vi "S4GUI_003.vi"(7 "Tab ObsEng":enum32{"Obs", "CCD modes", "Guider", "Eng"}(tab)) -> ()   [LabVIEW 2018] (continued)
            n1971 = local write "P15"(w3878) -> ()
            n1972 = call-dynamic "Write sequencia_ant.vi"("error in (no error)"=w3873, "sequencia_ant"=w3869, "Opt_Selector in"=w3875) -> ("error out"=w3872:errorcluster, "Opt_Selector out"=w3874:refnum<class "Opt_Selector.lvclass">)  [unwired: 7 in]
          }
          frame 2 {
            w3882 = u16 15 ("sequencia")
            w3891 = FALSE ("P0")
            w3892 = FALSE ("P0")
            w3893 = FALSE ("P0")
            w3894 = TRUE ("P0")
            # "0000 0000 0000 1111 = 15"
            n1973 = local write "P0"(w3894) -> ()
            n1974 = local write "P1"(w3894) -> ()
            n1975 = local write "P2"(w3894) -> ()
            n1976 = local write "P3"(w3894) -> ()
            n1977 = local write "P4"(w3892) -> ()
            n1978 = local write "P5"(w3892) -> ()
            n1979 = local write "P6"(w3892) -> ()
            n1980 = local write "P7"(w3892) -> ()
            n1981 = call-dynamic "Write sequencia.vi"("error in (no error)"=w3889, "sequencia"=w3882, "Opt_Selector in"=w3890) -> ("error out"=w3886:errorcluster, "Opt_Selector out"=w3888:refnum<class "Opt_Selector.lvclass">)  [unwired: 7 in]
            n1982 = call-dynamic "Write sequencia_ant.vi"("error in (no error)"=w3886, "sequencia_ant"=w3882, "Opt_Selector in"=w3888) -> ("error out"=w3885:errorcluster, "Opt_Selector out"=w3887:refnum<class "Opt_Selector.lvclass">)  [unwired: 7 in]
            n1983 = local write "P8"(w3893) -> ()
            n1984 = local write "P9"(w3893) -> ()
            n1985 = local write "P10"(w3893) -> ()
            n1986 = local write "P11"(w3893) -> ()
            n1987 = local write "P12"(w3891) -> ()
            n1988 = local write "P13"(w3891) -> ()
            n1989 = local write "P14"(w3891) -> ()
            n1990 = local write "P15"(w3891) -> ()
          }
          frame 3 {
            w3895 = u16 3855 ("sequencia")
            w3904 = FALSE ("P0")
            w3905 = FALSE ("P0")
            w3906 = TRUE ("P0")
            w3907 = TRUE ("P0")
            # "0000 1111 0000 1111 = 3855"
            n1991 = local write "P0"(w3907) -> ()
            n1992 = local write "P1"(w3907) -> ()
            n1993 = local write "P2"(w3907) -> ()
            n1994 = local write "P3"(w3907) -> ()
            n1995 = local write "P4"(w3905) -> ()
            n1996 = local write "P5"(w3905) -> ()
            n1997 = local write "P6"(w3905) -> ()
            n1998 = local write "P7"(w3905) -> ()
            n1999 = call-dynamic "Write sequencia.vi"("error in (no error)"=w3902, "sequencia"=w3895, "Opt_Selector in"=w3903) -> ("error out"=w3900:errorcluster, "Opt_Selector out"=w3901:refnum<class "Opt_Selector.lvclass">)  [unwired: 7 in]
            n2000 = local write "P8"(w3906) -> ()
            n2001 = local write "P9"(w3906) -> ()
            n2002 = local write "P10"(w3906) -> ()
            n2003 = local write "P11"(w3906) -> ()
            n2004 = local write "P12"(w3904) -> ()
            n2005 = local write "P13"(w3904) -> ()
            n2006 = local write "P14"(w3904) -> ()
            n2007 = local write "P15"(w3904) -> ()
            n2008 = call-dynamic "Write sequencia_ant.vi"("error in (no error)"=w3900, "sequencia_ant"=w3895, "Opt_Selector in"=w3901) -> ("error out"=w3899:errorcluster, "Opt_Selector out"=w3898:refnum<class "Opt_Selector.lvclass">)  [unwired: 7 in]
          }
          frame 4 {
            w3908 = u16 0 ("sequencia")
            w3917 = FALSE ("P0")
            w3918 = FALSE ("P0")
            w3919 = FALSE ("P0")
            w3920 = FALSE ("P0")
            n2009 = local write "P0"(w3920) -> ()
            n2010 = local write "P1"(w3920) -> ()
            n2011 = local write "P2"(w3920) -> ()
            n2012 = local write "P3"(w3920) -> ()
            n2013 = local write "P4"(w3918) -> ()
            n2014 = local write "P5"(w3918) -> ()
            n2015 = local write "P6"(w3918) -> ()
            n2016 = local write "P7"(w3918) -> ()
            n2017 = call-dynamic "Write sequencia.vi"("error in (no error)"=w3915, "sequencia"=w3908, "Opt_Selector in"=w3916) -> ("error out"=w3912:errorcluster, "Opt_Selector out"=w3914:refnum<class "Opt_Selector.lvclass">)  [unwired: 7 in]
            n2018 = call-dynamic "Write sequencia_ant.vi"("error in (no error)"=w3912, "sequencia_ant"=w3908, "Opt_Selector in"=w3914) -> ("error out"=w3911:errorcluster, "Opt_Selector out"=w3913:refnum<class "Opt_Selector.lvclass">)  [unwired: 7 in]
            n2019 = local write "P8"(w3919) -> ()
            n2020 = local write "P9"(w3919) -> ()
            n2021 = local write "P10"(w3919) -> ()
            n2022 = local write "P11"(w3919) -> ()
            n2023 = local write "P12"(w3917) -> ()
            n2024 = local write "P13"(w3917) -> ()
            n2025 = local write "P14"(w3917) -> ()
            n2026 = local write "P15"(w3917) -> ()
          }
          frame 5 {
            n2027 = call-dynamic "Read sequencia_ant.vi"("error in (no error)"=w3924, "Opt_Selector in"=w3925) -> ("error out"=w3923:errorcluster, "sequencia_ant"=w3921:u16, "Opt_Selector out"=w3922:refnum<class "Opt_Selector.lvclass">)  [unwired: 7 in]
          }
        }
        n2028 = call "Write WPROT.vi"("error in (no error)"=w3817, "Opt_Selector.lvclass"=w3824, "Instrument in"=w3823) -> ("error out"=w3826:errorcluster, "Instrument out"=w3827:refnum<class "Instrument.lvclass">)  [unwired: 7 in]
        n2029 = property on="#Pol. Seq. Done" class="Slide (strict)"(error in=w3817, "Scale.Maximum"=w3818, "Scale.Minimum"=w3816) -> ()  [unwired: 1 in, 2 out]
        n2030 = call "Write Instrument.lvclass.vi"("error in (no error)"=w3826, "Instrument.lvclass"=w3827, "S4ACS_GUI in"=w3822) -> ("error out"=w3806:errorcluster, "S4ACS_GUI out"=w3807:refnum<class "S4GUI.lvclass">)  [unwired: 7 in]
        n2031 = call "Read Instrument.lvclass.vi"("error in (no error)"=w3806, "S4ACS_GUI in"=w3807) -> ("error out"=w3811:errorcluster, "Instrument.lvclass"=w3812:refnum<class "Instrument.lvclass">, "S4ACS_GUI out"=w3815:refnum<class "S4GUI.lvclass">)  [unwired: 7 in]
        n2032 = call "Read ASEL.vi"("error in (no error)"=w3811, "Instrument in"=w3812) -> ("error out"=w3803:errorcluster, "Opt_Selector.lvclass"=w3805:refnum<class "Opt_Selector.lvclass">, "Instrument out"=w3808:refnum<class "Instrument.lvclass">)  [unwired: 7 in]
        n2033 = call "Read name_pos.vi"("error in (no error)"=w3803, "Optics in"=w3805) -> ("error out"=w3802:errorcluster, "name_pos"=w3801:string, "Optics out"=w3804:refnum<class "Opt_Selector.lvclass">)  [unwired: 7 in]
        n2034 = call "Write ASEL.vi"("error in (no error)"=w3802, "Opt_Selector.lvclass"=w3804, "Instrument in"=w3808) -> ("error out"=w3809:errorcluster, "Instrument out"=w3813:refnum<class "Instrument.lvclass">)  [unwired: 7 in]
        n2035 = case shown="\"ON\"" w3801 {
          tunnel: w3809 -> [w3832 w3843]
          tunnel: [w3832 w3839] -> w3810
          tunnel: w3813 -> [w3831 w3844]
          tunnel: [w3831 w3840] -> w3814
          frame Default {
          }
          frame "ON" {
            n2036 = call "Read WPROT.vi"("error in (no error)"=w3843, "Instrument in"=w3844) -> ("error out"=w3835:errorcluster, "Opt_Selector.lvclass"=w3842:refnum<class "Opt_Selector.lvclass">, "Instrument out"=w3841:refnum<class "Instrument.lvclass">)  [unwired: 7 in]
            n2037 = call-dynamic "Read sequencia.vi"("error in (no error)"=w3835, "Opt_Selector in"=w3842) -> ("error out"=w3834:errorcluster, "sequencia"=w3838:u16, "Opt_Selector out"=w3837:refnum<class "Opt_Selector.lvclass">)  [unwired: 7 in]
            n2038 = case shown="0" w3838 {
              tunnel: w3837 -> [w3846 w3855]
              tunnel: [w3846 w3851] -> w3836
              tunnel: w3834 -> [w3845 w3854]
              tunnel: [w3845 w3849] -> w3833
              frame Default {
              }
              frame 0 {
                n2039 = call-dynamic "Write sequencia.vi"("error in (no error)"=w3854, "sequencia"=u16 1, "Opt_Selector in"=w3855) -> ("error out"=w3850:errorcluster, "Opt_Selector out"=w3852:refnum<class "Opt_Selector.lvclass">)  [unwired: 7 in]
                n2040 = local write "P0"(TRUE ("P0")) -> ()
                n2041 = call-dynamic "Write sequencia_ant.vi"("error in (no error)"=w3850, "sequencia_ant"=u16 1, "Opt_Selector in"=w3852) -> ("error out"=w3849:errorcluster, "Opt_Selector out"=w3851:refnum<class "Opt_Selector.lvclass">)  [unwired: 7 in]
              }
            }
            n2042 = call "Write WPROT.vi"("error in (no error)"=w3833, "Opt_Selector.lvclass"=w3836, "Instrument in"=w3841) -> ("error out"=w3839:errorcluster, "Instrument out"=w3840:refnum<class "Instrument.lvclass">)  [unwired: 7 in]
          }
        }
        n2043 = call "Write Instrument.lvclass.vi"("error in (no error)"=w3810, "Instrument.lvclass"=w3814, "S4ACS_GUI in"=w3815) -> ("error out"=w3738:errorcluster, "S4ACS_GUI out"=w3739:refnum<class "S4GUI.lvclass">)  [unwired: 7 in]
        n2044 = call-dynamic "Read AcquisitionA.vi"("error in (no error)"=w3738, "S4ACS_GUI in"=w3739) -> ("error out"=w3798:errorcluster, "Acquisition.lvclass"=w3800:refnum<class "Acquisition.lvclass">, "S4ACS_GUI out"=w3797:refnum<class "S4GUI.lvclass">)  [unwired: 7 in]
        n2045 = call-dynamic "Read Channel.vi"("error in (no error)"=w3798, "Acquisition in"=w3800) -> ("error out"=w3794:errorcluster, "Channel.lvclass"=w3795:refnum<class "Channel.lvclass">, "Acquisition out"=w3799:refnum<class "Acquisition.lvclass">)  [unwired: 7 in]
        n2046 = call-dynamic "Write sequencias.vi"("error in (no error)"=w3794, "sequencias"=w3742, "Channel in"=w3795) -> ("error out"=w3791:errorcluster, "Channel out"=w3793:refnum<class "Channel.lvclass">)  [unwired: 7 in]
        n2047 = call-dynamic "Write prev sequencias.vi"("error in (no error)"=w3791, "prev sequencias"=w3742, "Channel in"=w3793) -> ("error out"=w3790:errorcluster, "Channel out"=w3792:refnum<class "Channel.lvclass">)  [unwired: 7 in]
        n2048 = call-dynamic "Write Channel.vi"("error in (no error)"=w3790, "Channel.lvclass"=w3792, "Acquisition in"=w3799) -> ("error out"=w3789:errorcluster, "Acquisition out"=w3796:refnum<class "Acquisition.lvclass">)  [unwired: 7 in]
        n2049 = call-dynamic "Write AcquisitionA.vi"("error in (no error)"=w3789, "Acquisition.lvclass"=w3796, "S4ACS_GUI in"=w3797) -> ("error out"=w3747:errorcluster, "S4ACS_GUI out"=w3748:refnum<class "S4GUI.lvclass">)  [unwired: 7 in]
        n2050 = call "Read AcquisitionB.vi"("error in (no error)"=w3747, "S4ACS_GUI in"=w3748) -> ("error out"=w3774:errorcluster, "Acquisition.lvclass"=w3776:refnum<class "Acquisition.lvclass">, "S4ACS_GUI out"=w3773:refnum<class "S4GUI.lvclass">)  [unwired: 7 in]
        n2051 = call-dynamic "Read Channel.vi"("error in (no error)"=w3774, "Acquisition in"=w3776) -> ("error out"=w3770:errorcluster, "Channel.lvclass"=w3771:refnum<class "Channel.lvclass">, "Acquisition out"=w3775:refnum<class "Acquisition.lvclass">)  [unwired: 7 in]
        n2052 = call-dynamic "Write sequencias.vi"("error in (no error)"=w3770, "sequencias"=w3742, "Channel in"=w3771) -> ("error out"=w3767:errorcluster, "Channel out"=w3769:refnum<class "Channel.lvclass">)  [unwired: 7 in]
        n2053 = call-dynamic "Write prev sequencias.vi"("error in (no error)"=w3767, "prev sequencias"=w3742, "Channel in"=w3769) -> ("error out"=w3766:errorcluster, "Channel out"=w3768:refnum<class "Channel.lvclass">)  [unwired: 7 in]
        n2054 = call-dynamic "Write Channel.vi"("error in (no error)"=w3766, "Channel.lvclass"=w3768, "Acquisition in"=w3775) -> ("error out"=w3765:errorcluster, "Acquisition out"=w3772:refnum<class "Acquisition.lvclass">)  [unwired: 7 in]
        n2055 = call "Write AcquisitionB.vi"("error in (no error)"=w3765, "Acquisition.lvclass"=w3772, "S4ACS_GUI in"=w3773) -> ("error out"=w3749:errorcluster, "S4ACS_GUI out"=w3750:refnum<class "S4GUI.lvclass">)  [unwired: 7 in]
        n2056 = call-dynamic "Read AcquisitionC.vi"("error in (no error)"=w3749, "S4ACS_GUI in"=w3750) -> ("error out"=w3762:errorcluster, "Acquisition.lvclass"=w3764:refnum<class "Acquisition.lvclass">, "S4ACS_GUI out"=w3761:refnum<class "S4GUI.lvclass">)  [unwired: 7 in]
        n2057 = call-dynamic "Read Channel.vi"("error in (no error)"=w3762, "Acquisition in"=w3764) -> ("error out"=w3758:errorcluster, "Channel.lvclass"=w3759:refnum<class "Channel.lvclass">, "Acquisition out"=w3763:refnum<class "Acquisition.lvclass">)  [unwired: 7 in]
        n2058 = call-dynamic "Write sequencias.vi"("error in (no error)"=w3758, "sequencias"=w3742, "Channel in"=w3759) -> ("error out"=w3755:errorcluster, "Channel out"=w3757:refnum<class "Channel.lvclass">)  [unwired: 7 in]
        n2059 = call-dynamic "Write prev sequencias.vi"("error in (no error)"=w3755, "prev sequencias"=w3742, "Channel in"=w3757) -> ("error out"=w3754:errorcluster, "Channel out"=w3756:refnum<class "Channel.lvclass">)  [unwired: 7 in]
        n2060 = call-dynamic "Write Channel.vi"("error in (no error)"=w3754, "Channel.lvclass"=w3756, "Acquisition in"=w3763) -> ("error out"=w3753:errorcluster, "Acquisition out"=w3760:refnum<class "Acquisition.lvclass">)  [unwired: 7 in]
        n2061 = call-dynamic "Write AcquisitionC.vi"("error in (no error)"=w3753, "Acquisition.lvclass"=w3760, "S4ACS_GUI in"=w3761) -> ("error out"=w3745:errorcluster, "S4ACS_GUI out"=w3746:refnum<class "S4GUI.lvclass">)  [unwired: 7 in]
        n2062 = call-dynamic "Read AcquisitionD.vi"("error in (no error)"=w3745, "S4ACS_GUI in"=w3746) -> ("error out"=w3786:errorcluster, "Acquisition.lvclass"=w3788:refnum<class "Acquisition.lvclass">, "S4ACS_GUI out"=w3785:refnum<class "S4GUI.lvclass">)  [unwired: 7 in]
        n2063 = call-dynamic "Read Channel.vi"("error in (no error)"=w3786, "Acquisition in"=w3788) -> ("error out"=w3782:errorcluster, "Channel.lvclass"=w3783:refnum<class "Channel.lvclass">, "Acquisition out"=w3787:refnum<class "Acquisition.lvclass">)  [unwired: 7 in]
        n2064 = call-dynamic "Write sequencias.vi"("error in (no error)"=w3782, "sequencias"=w3742, "Channel in"=w3783) -> ("error out"=w3779:errorcluster, "Channel out"=w3781:refnum<class "Channel.lvclass">)  [unwired: 7 in]
        n2065 = call-dynamic "Write prev sequencias.vi"("error in (no error)"=w3779, "prev sequencias"=w3742, "Channel in"=w3781) -> ("error out"=w3778:errorcluster, "Channel out"=w3780:refnum<class "Channel.lvclass">)  [unwired: 7 in]
        n2066 = call-dynamic "Write Channel.vi"("error in (no error)"=w3778, "Channel.lvclass"=w3780, "Acquisition in"=w3787) -> ("error out"=w3777:errorcluster, "Acquisition out"=w3784:refnum<class "Acquisition.lvclass">)  [unwired: 7 in]
        n2067 = call-dynamic "Write AcquisitionD.vi"("error in (no error)"=w3777, "Acquisition.lvclass"=w3784, "S4ACS_GUI in"=w3785) -> ("error out"=w3743:errorcluster, "S4ACS_GUI out"=w3744:refnum<class "S4GUI.lvclass">)  [unwired: 7 in]
        n2068 = call-dynamic "Write sequencias.vi"("error in (no error)"=w3743, "sequencias"=w3742, "S4GUI in"=w3744) -> ("error out"=w3752:errorcluster, "S4GUI out"=w3751:refnum<class "S4GUI.lvclass">)  [unwired: 7 in]
        n2069 = call-dynamic "Write prev sequencias.vi"("error in (no error)"=w3752, "prev sequencias"=w3742, "S4GUI in"=w3751) -> ("error out"=w3740:errorcluster, "S4GUI out"=w3741:refnum<class "S4GUI.lvclass">)  [unwired: 7 in]
      }
      event "P0", "P1", "P2", "P3", "P4", "P5", "P6", "P7", "P8", "P9", "P10", "P11", "P12", "P13", "P14", "P15": Value Change {
        w4041 = u16 5 items=["All 16 positions", "First 8 positions", "First 4 positions", "0-3 + 8-11", "Clear", "Customized"] ("Select Positions")
        # "Garantir que, quando em POLARIMETRIA, pelo menos WP1 esteja selecionado."
        # "Salva tambem em \nSequencia_ant para\no caso de repeticao."
        n2070 = event-data() -> ()  [unwired: 1 in, 6 out]
        n2071 = local write "Select Positions"(w4041) -> ()
        n2072 = call "Read Instrument.lvclass.vi"("error in (no error)"=w4023, "S4ACS_GUI in"=w4024) -> ("error out"=w4018:errorcluster, "Instrument.lvclass"=w4021:refnum<class "Instrument.lvclass">, "S4ACS_GUI out"=w4022:refnum<class "S4GUI.lvclass">)  [unwired: 7 in]
        n2073 = Build Array("P0", "P1", "P2", "P3", "P4", "P5", "P6", "P7", "P8", "P9", "P10", "P11", "P12", "P13", "P14", "P15") -> (w4010:bool[])
        n2074 = call "Read WPROT.vi"("error in (no error)"=w4018, "Instrument in"=w4021) -> ("error out"=w4017:errorcluster, "Opt_Selector.lvclass"=w4019:refnum<class "Opt_Selector.lvclass">, "Instrument out"=w4020:refnum<class "Instrument.lvclass">)  [unwired: 7 in]
        n2075 = Boolean Array To Number(Boolean array=w4010) -> (number=w4025:u32)
        n2076 = To Unsigned Word Integer(number=w4025) -> (unsigned 16bit integer=w3928:u16)
        n2077 = call-dynamic "Write sequencia.vi"("error in (no error)"=w4017, "sequencia"=w3928, "Opt_Selector in"=w4019) -> ("error out"=w4012:errorcluster, "Opt_Selector out"=w4014:refnum<class "Opt_Selector.lvclass">)  [unwired: 7 in]
        n2078 = call-dynamic "Write sequencia_ant.vi"("error in (no error)"=w4012, "sequencia_ant"=w3928, "Opt_Selector in"=w4014) -> ("error out"=w4011:errorcluster, "Opt_Selector out"=w4013:refnum<class "Opt_Selector.lvclass">)  [unwired: 7 in]
        n2079 = call "Write WPROT.vi"("error in (no error)"=w4011, "Opt_Selector.lvclass"=w4013, "Instrument in"=w4020) -> ("error out"=w4016:errorcluster, "Instrument out"=w4015:refnum<class "Instrument.lvclass">)  [unwired: 7 in]
        n2080 = call "Write Instrument.lvclass.vi"("error in (no error)"=w4016, "Instrument.lvclass"=w4015, "S4ACS_GUI in"=w4022) -> ("error out"=w3991:errorcluster, "S4ACS_GUI out"=w3992:refnum<class "S4GUI.lvclass">)  [unwired: 7 in]
        n2081 = call "Read Instrument.lvclass.vi"("error in (no error)"=w3991, "S4ACS_GUI in"=w3992) -> ("error out"=w3997:errorcluster, "Instrument.lvclass"=w3996:refnum<class "Instrument.lvclass">, "S4ACS_GUI out"=w3993:refnum<class "S4GUI.lvclass">)  [unwired: 7 in]
        n2082 = call "Read ASEL.vi"("error in (no error)"=w3997, "Instrument in"=w3996) -> ("error out"=w4003:errorcluster, "Opt_Selector.lvclass"=w4001:refnum<class "Opt_Selector.lvclass">, "Instrument out"=w4000:refnum<class "Instrument.lvclass">)  [unwired: 7 in]
        n2083 = call "Read name_pos.vi"("error in (no error)"=w4003, "Optics in"=w4001) -> ("error out"=w4004:errorcluster, "name_pos"=w4005:string, "Optics out"=w4002:refnum<class "Opt_Selector.lvclass">)  [unwired: 7 in]
        n2084 = call "Write ASEL.vi"("error in (no error)"=w4004, "Opt_Selector.lvclass"=w4002, "Instrument in"=w4000) -> ("error out"=w3999:errorcluster, "Instrument out"=w3995:refnum<class "Instrument.lvclass">)  [unwired: 7 in]
        n2085 = case shown="\"ON\"" w4005 {
          tunnel: w3999 -> [w4043 w4054]
          tunnel: [w4043 w4050] -> w3998
          tunnel: w3995 -> [w4042 w4055]
          tunnel: [w4042 w4051] -> w3994
          frame Default {
          }
          frame "ON" {
            n2086 = call "Read WPROT.vi"("error in (no error)"=w4054, "Instrument in"=w4055) -> ("error out"=w4046:errorcluster, "Opt_Selector.lvclass"=w4053:refnum<class "Opt_Selector.lvclass">, "Instrument out"=w4052:refnum<class "Instrument.lvclass">)  [unwired: 7 in]
            n2087 = call-dynamic "Read sequencia.vi"("error in (no error)"=w4046, "Opt_Selector in"=w4053) -> ("error out"=w4045:errorcluster, "sequencia"=w4049:u16, "Opt_Selector out"=w4048:refnum<class "Opt_Selector.lvclass">)  [unwired: 7 in]
            n2088 = case shown="0" w4049 {
              tunnel: w4048 -> [w4057 w4066]
              tunnel: [w4057 w4062] -> w4047
              tunnel: w4045 -> [w4056 w4065]
              tunnel: [w4056 w4060] -> w4044
              frame Default {
              }
              frame 0 {
                n2089 = call-dynamic "Write sequencia.vi"("error in (no error)"=w4065, "sequencia"=u16 1, "Opt_Selector in"=w4066) -> ("error out"=w4061:errorcluster, "Opt_Selector out"=w4063:refnum<class "Opt_Selector.lvclass">)  [unwired: 7 in]
                n2090 = local write "P0"(TRUE ("P0")) -> ()
                n2091 = call-dynamic "Write sequencia_ant.vi"("error in (no error)"=w4061, "sequencia_ant"=u16 1, "Opt_Selector in"=w4063) -> ("error out"=w4060:errorcluster, "Opt_Selector out"=w4062:refnum<class "Opt_Selector.lvclass">)  [unwired: 7 in]
              }
            }
            n2092 = call "Write WPROT.vi"("error in (no error)"=w4044, "Opt_Selector.lvclass"=w4047, "Instrument in"=w4052) -> ("error out"=w4050:errorcluster, "Instrument out"=w4051:refnum<class "Instrument.lvclass">)  [unwired: 7 in]
          }
        }
        n2093 = for {
          tunnel: w4010 -> [w4070] mode=indexing
          shift-right: [w4069] -> w4008
          shift-left: 0 -> [w4067]
          # "calcula qtd de 1s"
          n2094 = Increment(x=w4067) -> (x+1=w4068:i32)
          n2095 = Select(t=w4068, s=w4070, f=w4067) -> (s? t:f=w4069:i32)
        }
        n2096 = property on="#Pol. Seq. Done" class="Slide (strict)"("Scale.Maximum"=w4008, "Scale.Minimum"=0.0 ("Scale.Range:Minimum")) -> ()  [unwired: 2 in, 2 out]
        n2097 = call "Write Instrument.lvclass.vi"("error in (no error)"=w3998, "Instrument.lvclass"=w3994, "S4ACS_GUI in"=w3993) -> ("error out"=w3935:errorcluster, "S4ACS_GUI out"=w3936:refnum<class "S4GUI.lvclass">)  [unwired: 7 in]
        n2098 = call-dynamic "Read AcquisitionA.vi"("error in (no error)"=w3935, "S4ACS_GUI in"=w3936) -> ("error out"=w3988:errorcluster, "Acquisition.lvclass"=w3990:refnum<class "Acquisition.lvclass">, "S4ACS_GUI out"=w3987:refnum<class "S4GUI.lvclass">)  [unwired: 7 in]
        n2099 = call-dynamic "Read Channel.vi"("error in (no error)"=w3988, "Acquisition in"=w3990) -> ("error out"=w3984:errorcluster, "Channel.lvclass"=w3985:refnum<class "Channel.lvclass">, "Acquisition out"=w3989:refnum<class "Acquisition.lvclass">)  [unwired: 7 in]
        n2100 = call-dynamic "Write sequencias.vi"("error in (no error)"=w3984, "sequencias"=w3928, "Channel in"=w3985) -> ("error out"=w3981:errorcluster, "Channel out"=w3983:refnum<class "Channel.lvclass">)  [unwired: 7 in]
        n2101 = call-dynamic "Write prev sequencias.vi"("error in (no error)"=w3981, "prev sequencias"=w3928, "Channel in"=w3983) -> ("error out"=w3980:errorcluster, "Channel out"=w3982:refnum<class "Channel.lvclass">)  [unwired: 7 in]
        n2102 = call-dynamic "Write Channel.vi"("error in (no error)"=w3980, "Channel.lvclass"=w3982, "Acquisition in"=w3989) -> ("error out"=w3979:errorcluster, "Acquisition out"=w3986:refnum<class "Acquisition.lvclass">)  [unwired: 7 in]
        n2103 = call-dynamic "Write AcquisitionA.vi"("error in (no error)"=w3979, "Acquisition.lvclass"=w3986, "S4ACS_GUI in"=w3987) -> ("error out"=w3933:errorcluster, "S4ACS_GUI out"=w3934:refnum<class "S4GUI.lvclass">)  [unwired: 7 in]
        n2104 = call "Read AcquisitionB.vi"("error in (no error)"=w3933, "S4ACS_GUI in"=w3934) -> ("error out"=w3964:errorcluster, "Acquisition.lvclass"=w3966:refnum<class "Acquisition.lvclass">, "S4ACS_GUI out"=w3963:refnum<class "S4GUI.lvclass">)  [unwired: 7 in]
        n2105 = call-dynamic "Read Channel.vi"("error in (no error)"=w3964, "Acquisition in"=w3966) -> ("error out"=w3960:errorcluster, "Channel.lvclass"=w3961:refnum<class "Channel.lvclass">, "Acquisition out"=w3965:refnum<class "Acquisition.lvclass">)  [unwired: 7 in]
        n2106 = call-dynamic "Write sequencias.vi"("error in (no error)"=w3960, "sequencias"=w3928, "Channel in"=w3961) -> ("error out"=w3957:errorcluster, "Channel out"=w3959:refnum<class "Channel.lvclass">)  [unwired: 7 in]
        n2107 = call-dynamic "Write prev sequencias.vi"("error in (no error)"=w3957, "prev sequencias"=w3928, "Channel in"=w3959) -> ("error out"=w3956:errorcluster, "Channel out"=w3958:refnum<class "Channel.lvclass">)  [unwired: 7 in]
        n2108 = call-dynamic "Write Channel.vi"("error in (no error)"=w3956, "Channel.lvclass"=w3958, "Acquisition in"=w3965) -> ("error out"=w3955:errorcluster, "Acquisition out"=w3962:refnum<class "Acquisition.lvclass">)  [unwired: 7 in]
        n2109 = call "Write AcquisitionB.vi"("error in (no error)"=w3955, "Acquisition.lvclass"=w3962, "S4ACS_GUI in"=w3963) -> ("error out"=w3937:errorcluster, "S4ACS_GUI out"=w3938:refnum<class "S4GUI.lvclass">)  [unwired: 7 in]
        n2110 = call-dynamic "Read AcquisitionC.vi"("error in (no error)"=w3937, "S4ACS_GUI in"=w3938) -> ("error out"=w3952:errorcluster, "Acquisition.lvclass"=w3954:refnum<class "Acquisition.lvclass">, "S4ACS_GUI out"=w3951:refnum<class "S4GUI.lvclass">)  [unwired: 7 in]
        n2111 = call-dynamic "Read Channel.vi"("error in (no error)"=w3952, "Acquisition in"=w3954) -> ("error out"=w3948:errorcluster, "Channel.lvclass"=w3949:refnum<class "Channel.lvclass">, "Acquisition out"=w3953:refnum<class "Acquisition.lvclass">)  [unwired: 7 in]
        n2112 = call-dynamic "Write sequencias.vi"("error in (no error)"=w3948, "sequencias"=w3928, "Channel in"=w3949) -> ("error out"=w3945:errorcluster, "Channel out"=w3947:refnum<class "Channel.lvclass">)  [unwired: 7 in]
        n2113 = call-dynamic "Write prev sequencias.vi"("error in (no error)"=w3945, "prev sequencias"=w3928, "Channel in"=w3947) -> ("error out"=w3944:errorcluster, "Channel out"=w3946:refnum<class "Channel.lvclass">)  [unwired: 7 in]
        n2114 = call-dynamic "Write Channel.vi"("error in (no error)"=w3944, "Channel.lvclass"=w3946, "Acquisition in"=w3953) -> ("error out"=w3943:errorcluster, "Acquisition out"=w3950:refnum<class "Acquisition.lvclass">)  [unwired: 7 in]
        n2115 = call-dynamic "Write AcquisitionC.vi"("error in (no error)"=w3943, "Acquisition.lvclass"=w3950, "S4ACS_GUI in"=w3951) -> ("error out"=w3931:errorcluster, "S4ACS_GUI out"=w3932:refnum<class "S4GUI.lvclass">)  [unwired: 7 in]
        n2116 = call-dynamic "Read AcquisitionD.vi"("error in (no error)"=w3931, "S4ACS_GUI in"=w3932) -> ("error out"=w3976:errorcluster, "Acquisition.lvclass"=w3978:refnum<class "Acquisition.lvclass">, "S4ACS_GUI out"=w3975:refnum<class "S4GUI.lvclass">)  [unwired: 7 in]
        n2117 = call-dynamic "Read Channel.vi"("error in (no error)"=w3976, "Acquisition in"=w3978) -> ("error out"=w3972:errorcluster, "Channel.lvclass"=w3973:refnum<class "Channel.lvclass">, "Acquisition out"=w3977:refnum<class "Acquisition.lvclass">)  [unwired: 7 in]
        n2118 = call-dynamic "Write sequencias.vi"("error in (no error)"=w3972, "sequencias"=w3928, "Channel in"=w3973) -> ("error out"=w3969:errorcluster, "Channel out"=w3971:refnum<class "Channel.lvclass">)  [unwired: 7 in]
        n2119 = call-dynamic "Write prev sequencias.vi"("error in (no error)"=w3969, "prev sequencias"=w3928, "Channel in"=w3971) -> ("error out"=w3968:errorcluster, "Channel out"=w3970:refnum<class "Channel.lvclass">)  [unwired: 7 in]
        n2120 = call-dynamic "Write Channel.vi"("error in (no error)"=w3968, "Channel.lvclass"=w3970, "Acquisition in"=w3977) -> ("error out"=w3967:errorcluster, "Acquisition out"=w3974:refnum<class "Acquisition.lvclass">)  [unwired: 7 in]
        n2121 = call-dynamic "Write AcquisitionD.vi"("error in (no error)"=w3967, "Acquisition.lvclass"=w3974, "S4ACS_GUI in"=w3975) -> ("error out"=w3929:errorcluster, "S4ACS_GUI out"=w3930:refnum<class "S4GUI.lvclass">)  [unwired: 7 in]
        n2122 = call-dynamic "Write sequencias.vi"("error in (no error)"=w3929, "sequencias"=w3928, "S4GUI in"=w3930) -> ("error out"=w3941:errorcluster, "S4GUI out"=w3940:refnum<class "S4GUI.lvclass">)  [unwired: 7 in]
        n2123 = call-dynamic "Write prev sequencias.vi"("error in (no error)"=w3941, "prev sequencias"=w3928, "S4GUI in"=w3940) -> ("error out"=w3942:errorcluster, "S4GUI out"=w3939:refnum<class "S4GUI.lvclass">)  [unwired: 7 in]
      }
      event "SSM": Value Change {
        # "F: fotom.\nT: polar."
        n2124 = event-data() -> ("NewVal"=w4078:u16)  [unwired: 1 in, 5 out]
        n2125 = call-dynamic "Read mode EXPOSE.vi"("error in (no error)"=w4084, "S4GUI in"=w4085) -> ("error out"=w4083:errorcluster, "mode EXPOSE"=w4079:bool, "S4GUI out"=w4080:refnum<class "S4GUI.lvclass">)  [unwired: 7 in]
        n2126 = call "Read Instrument.lvclass.vi"("error in (no error)"=w4083, "S4ACS_GUI in"=w4080) -> ("error out"=w4082:errorcluster, "Instrument.lvclass"=w4088:refnum<class "Instrument.lvclass">, "S4ACS_GUI out"=w4087:refnum<class "S4GUI.lvclass">)  [unwired: 7 in]
        n2127 = call-dynamic "Read mode.vi"("error in (no error)"=w4082, "Instrument in"=w4088) -> ("error out"=w4081:errorcluster, "mode"=w4086:bool)  [unwired: 7 in, 1 out]
        n2128 = case shown="1" w4078 {
          tunnel: [TRUE FALSE] -> w4091
          tunnel: w4081 -> [w4102 w4328]
          tunnel: w4087 -> [w4104 w4327]
          tunnel: [w4095 w4319] -> w4090
          tunnel: [w4094 w4318] -> w4089
          tunnel: w4086 -> [_ w4308]
          tunnel: w4079 -> [_ w4306]
          tunnel: ["SYNCHRONOUS" "ASYNCHRONOUS"] -> w4071
          frame 1 {
            # "Sync mode: Os canais sao configurados para Trigger externo, desde que o SyncBox esteja conectado."
            # "Sync by Cycle"
            n2129 = call-dynamic "Read Sync Box.lvclass.vi"("error in (no error)"=w4102, "SPARC4_AC in"=w4104) -> ("error out"=w4101:errorcluster, "Sync Box.lvclass"=w4105:refnum<class "Sync Box.lvclass">, "SPARC4_AC out"=w4103:refnum<class "S4GUI.lvclass">)  [unwired: 7 in]
            n2130 = call "Read connection.vi"("error in (no error)"=w4101, "Server in"=w4105) -> ("error out"=w4100:errorcluster, "connection"=w4099:bool)  [unwired: 7 in, 1 out]
            n2131 = case shown="False" w4099 {
              tunnel: [w4108 w4125] -> w4097
              tunnel: w4103 -> [w4108 w4115]
              tunnel: w4100 -> [w4107 w4114]
              tunnel: [w4107 w4109] -> w4096
              frame False {
              }
              frame True {
                n2132 = call-dynamic "Read AcquisitionC.vi"("error in (no error)"=w4114, "S4ACS_GUI in"=w4115) -> ("error out"=w4132:errorcluster, "Acquisition.lvclass"=w4131:refnum<class "Acquisition.lvclass">)  [unwired: 7 in, 1 out]
                n2133 = call-dynamic "Read AcquisitionA.vi"("error in (no error)"=w4114, "S4ACS_GUI in"=w4115) -> ("error out"=w4135:errorcluster, "Acquisition.lvclass"=w4136:refnum<class "Acquisition.lvclass">, "S4ACS_GUI out"=w4124:refnum<class "S4GUI.lvclass">)  [unwired: 7 in]
                n2134 = call "Read AcquisitionB.vi"("error in (no error)"=w4114, "S4ACS_GUI in"=w4115) -> ("error out"=w4133:errorcluster, "Acquisition.lvclass"=w4134:refnum<class "Acquisition.lvclass">)  [unwired: 7 in, 1 out]
                n2135 = call-dynamic "Read AcquisitionD.vi"("error in (no error)"=w4114, "S4ACS_GUI in"=w4115) -> ("error out"=w4129:errorcluster, "Acquisition.lvclass"=w4130:refnum<class "Acquisition.lvclass">)  [unwired: 7 in, 1 out]
                n2136 = call-dynamic "Read enabled.vi"("error in (no error)"=w4129, "Server in"=w4130) -> ("error out"=w4138:errorcluster, "enabled"=w4137:bool, "Server out"=w4139:refnum<class "Acquisition.lvclass">)  [unwired: 7 in]
                n2137 = call-dynamic "Read enabled.vi"("error in (no error)"=w4132, "Server in"=w4131) -> ("error out"=w4141:errorcluster, "enabled"=w4140:bool, "Server out"=w4142:refnum<class "Acquisition.lvclass">)  [unwired: 7 in]
                n2138 = call-dynamic "Read enabled.vi"("error in (no error)"=w4133, "Server in"=w4134) -> ("error out"=w4144:errorcluster, "enabled"=w4143:bool, "Server out"=w4145:refnum<class "Acquisition.lvclass">)  [unwired: 7 in]
                n2139 = call-dynamic "Read enabled.vi"("error in (no error)"=w4135, "Server in"=w4136) -> ("error out"=w4147:errorcluster, "enabled"=w4146:bool, "Server out"=w4148:refnum<class "Acquisition.lvclass">)  [unwired: 7 in]
                n2140 = case shown="True" w4143 {
                  tunnel: w4145 -> [w4228 w4232]
                  tunnel: w4144 -> [w4227 w4231]
                  tunnel: [w4228 w4230] -> w4121
                  tunnel: [w4227 w4229] -> w4120
                  frame False {
                  }
                  frame True {
                    # "Ext Start"
                    # "nome do arquivo .cfg"
                    # "seção no arquivo .cfg"
                    n2141 = call-dynamic "Read Channel.vi"("error in (no error)"=w4231, "Acquisition in"=w4232) -> ("error out"=w4236:errorcluster, "Channel.lvclass"=w4235:refnum<class "Channel.lvclass">, "Acquisition out"=w4234:refnum<class "Acquisition.lvclass">)  [unwired: 7 in]
                    n2142 = call-dynamic "Read Interface.vi"("error in (no error)"=w4236, "Channel in"=w4235) -> ("error out"=w4244:errorcluster, "Interface.lvclass"=w4245:refnum<class "Interface.lvclass">, "Channel out"=w4233:refnum<class "Channel.lvclass">)  [unwired: 7 in]
                    n2143 = call-dynamic "Get CCD_Config.vi"("error in (no error)"=w4244, "Interface in"=w4245) -> ("error out"=w4241:errorcluster, "output cluster"=w4240:T31, "Interface out"=w4246:refnum<class "Interface.lvclass">)  [unwired: 7 in]
                    n2144 = Bundle By Name(cluster=w4240, "TRIGGER_MODE"=u8 6 ("SHUTTER_MODE")) -> (w4242:T31)
                    n2145 = call-dynamic "Set CCD_Config.vi"("error in (no error)"=w4241, "input cluster"=w4242, "Interface in"=w4246) -> ("error out"=w4239:errorcluster, "Interface out"=w4247:refnum<class "Interface.lvclass">)  [unwired: 7 in]
                    n2146 = Flatten To String(anything=w4242, error in (no error)=w4239) -> (data string=w4237:string, error out=w4238:errorcluster)  [unwired: 2 in, 1 out]
                    n2147 = call "Write flatted cluster.vi"("error in (no error)"=w4238, "flatted cluster"=w4237, "Interface in"=w4247) -> ("error out"=w4249:errorcluster, "Interface out"=w4248:refnum<class "Interface.lvclass">)  [unwired: 7 in]
                    n2148 = call-dynamic "Write Interface.vi"("error in (no error)"=w4249, "Interface.lvclass"=w4248, "Channel in"=w4233) -> ("error out"=w4255:errorcluster, "Channel out"=w4256:refnum<class "Channel.lvclass">)  [unwired: 7 in]
                    n2149 = call "Write section_name.vi"("error in (no error)"=w4255, "section_name"="CCD_ACS2", "Channel in"=w4256) -> ("error out"=w4253:errorcluster, "Channel out"=w4259:refnum<class "Channel.lvclass">)  [unwired: 7 in]
                    n2150 = call-dynamic "save config.vi"("error in (no error)"=w4253, "file config"="lastsaved.cfg", "Channel in"=w4259) -> ("error out"=w4254:errorcluster, "Channel out"=w4260:refnum<class "Channel.lvclass">)  [unwired: 7 in]
                    n2151 = call-dynamic "Read State Machine.vi"("error in (no error)"=w4254, "Device in"=w4260) -> ("error out"=w4250:errorcluster, "State Machine.lvclass"=w4262:refnum<class "State Machine.lvclass">, "Device out"=w4261:refnum<class "Channel.lvclass">)  [unwired: 7 in]
                    n2152 = call-dynamic "Write State.vi"("error in (no error)"=w4250, "State"=60, "State Machine in"=w4262) -> ("error out"=w4251:errorcluster, "State Machine out"=w4263:refnum<class "State Machine.lvclass">)  [unwired: 7 in]
                    n2153 = call-dynamic "Write State Machine.vi"("error in (no error)"=w4251, "State Machine.lvclass"=w4263, "Device in"=w4261) -> ("error out"=w4265:errorcluster, "Device out"=w4264:refnum<class "Channel.lvclass">)  [unwired: 7 in]
                    n2154 = call-dynamic "Write Channel.vi"("error in (no error)"=w4265, "Channel.lvclass"=w4264, "Acquisition in"=w4234) -> ("error out"=w4229:errorcluster, "Acquisition out"=w4230:refnum<class "Acquisition.lvclass">)  [unwired: 7 in]
                  }
                }
                n2155 = case shown="True" w4146 {
                  tunnel: [w4266 w4300] -> w4122
                  tunnel: [w4267 w4299] -> w4123
                  tunnel: w4148 -> [w4267 w4269]
                  tunnel: w4147 -> [w4266 w4268]
                  frame False {
                  }
                  frame True {
                    # "nome do arquivo .cfg"
                    # "seção no arquivo .cfg"
                    # "Ext Start"
                    n2156 = call-dynamic "Read Channel.vi"("error in (no error)"=w4268, "Acquisition in"=w4269) -> ("error out"=w4301:errorcluster, "Channel.lvclass"=w4302:refnum<class "Channel.lvclass">, "Acquisition out"=w4303:refnum<class "Acquisition.lvclass">)  [unwired: 7 in]
                    n2157 = call-dynamic "Read Interface.vi"("error in (no error)"=w4301, "Channel in"=w4302) -> ("error out"=w4291:errorcluster, "Interface.lvclass"=w4290:refnum<class "Interface.lvclass">, "Channel out"=w4304:refnum<class "Channel.lvclass">)  [unwired: 7 in]
                    n2158 = call-dynamic "Get CCD_Config.vi"("error in (no error)"=w4291, "Interface in"=w4290) -> ("error out"=w4294:errorcluster, "output cluster"=w4295:T31, "Interface out"=w4289:refnum<class "Interface.lvclass">)  [unwired: 7 in]
                    n2159 = Bundle By Name(cluster=w4295, "TRIGGER_MODE"=u8 6 ("SHUTTER_MODE")) -> (w4293:T31)
                    n2160 = call-dynamic "Set CCD_Config.vi"("error in (no error)"=w4294, "input cluster"=w4293, "Interface in"=w4289) -> ("error out"=w4296:errorcluster, "Interface out"=w4288:refnum<class "Interface.lvclass">)  [unwired: 7 in]
                    n2161 = Flatten To String(anything=w4293, error in (no error)=w4296) -> (data string=w4298:string, error out=w4297:errorcluster)  [unwired: 2 in, 1 out]
                    n2162 = call "Write flatted cluster.vi"("error in (no error)"=w4297, "flatted cluster"=w4298, "Interface in"=w4288) -> ("error out"=w4286:errorcluster, "Interface out"=w4287:refnum<class "Interface.lvclass">)  [unwired: 7 in]
                    n2163 = call-dynamic "Write Interface.vi"("error in (no error)"=w4286, "Interface.lvclass"=w4287, "Channel in"=w4304) -> ("error out"=w4281:errorcluster, "Channel out"=w4280:refnum<class "Channel.lvclass">)  [unwired: 7 in]
                    n2164 = call "Write section_name.vi"("error in (no error)"=w4281, "section_name"="CCD_ACS1", "Channel in"=w4280) -> ("error out"=w4282:errorcluster, "Channel out"=w4277:refnum<class "Channel.lvclass">)  [unwired: 7 in]
                    n2165 = call-dynamic "save config.vi"("error in (no error)"=w4282, "file config"="lastsaved.cfg", "Channel in"=w4277) -> ("error out"=w4270:errorcluster, "Channel out"=w4271:refnum<class "Channel.lvclass">)  [unwired: 7 in]
                    n2166 = call-dynamic "Read State Machine.vi"("error in (no error)"=w4270, "Device in"=w4271) -> ("error out"=w4285:errorcluster, "State Machine.lvclass"=w4275:refnum<class "State Machine.lvclass">, "Device out"=w4276:refnum<class "Channel.lvclass">)  [unwired: 7 in]
                    n2167 = call-dynamic "Write State.vi"("error in (no error)"=w4285, "State"=60, "State Machine in"=w4275) -> ("error out"=w4284:errorcluster, "State Machine out"=w4274:refnum<class "State Machine.lvclass">)  [unwired: 7 in]
                    n2168 = call-dynamic "Write State Machine.vi"("error in (no error)"=w4284, "State Machine.lvclass"=w4274, "Device in"=w4276) -> ("error out"=w4272:errorcluster, "Device out"=w4273:refnum<class "Channel.lvclass">)  [unwired: 7 in]
                    n2169 = call-dynamic "Write Channel.vi"("error in (no error)"=w4272, "Channel.lvclass"=w4273, "Acquisition in"=w4303) -> ("error out"=w4300:errorcluster, "Acquisition out"=w4299:refnum<class "Acquisition.lvclass">)  [unwired: 7 in]
                  }
                }
                n2170 = case shown="True" w4140 {
                  tunnel: w4142 -> [w4189 w4193]
                  tunnel: w4141 -> [w4188 w4192]
                  tunnel: [w4189 w4191] -> w4119
                  tunnel: [w4188 w4190] -> w4118
                  frame False {
                  }
                  frame True {
                    # "Ext Start"
                    # "nome do arquivo .cfg"
                    # "seção no arquivo .cfg"
                    n2171 = call-dynamic "Read Channel.vi"("error in (no error)"=w4192, "Acquisition in"=w4193) -> ("error out"=w4197:errorcluster, "Channel.lvclass"=w4196:refnum<class "Channel.lvclass">, "Acquisition out"=w4195:refnum<class "Acquisition.lvclass">)  [unwired: 7 in]
                    n2172 = call-dynamic "Read Interface.vi"("error in (no error)"=w4197, "Channel in"=w4196) -> ("error out"=w4205:errorcluster, "Interface.lvclass"=w4206:refnum<class "Interface.lvclass">, "Channel out"=w4194:refnum<class "Channel.lvclass">)  [unwired: 7 in]
                    n2173 = call-dynamic "Get CCD_Config.vi"("error in (no error)"=w4205, "Interface in"=w4206) -> ("error out"=w4202:errorcluster, "output cluster"=w4201:T31, "Interface out"=w4207:refnum<class "Interface.lvclass">)  [unwired: 7 in]
                    n2174 = Bundle By Name(cluster=w4201, "TRIGGER_MODE"=u8 6 ("SHUTTER_MODE")) -> (w4203:T31)
                    n2175 = call-dynamic "Set CCD_Config.vi"("error in (no error)"=w4202, "input cluster"=w4203, "Interface in"=w4207) -> ("error out"=w4200:errorcluster, "Interface out"=w4208:refnum<class "Interface.lvclass">)  [unwired: 7 in]
                    n2176 = Flatten To String(anything=w4203, error in (no error)=w4200) -> (data string=w4198:string, error out=w4199:errorcluster)  [unwired: 2 in, 1 out]
                    n2177 = call "Write flatted cluster.vi"("error in (no error)"=w4199, "flatted cluster"=w4198, "Interface in"=w4208) -> ("error out"=w4210:errorcluster, "Interface out"=w4209:refnum<class "Interface.lvclass">)  [unwired: 7 in]
                    n2178 = call-dynamic "Write Interface.vi"("error in (no error)"=w4210, "Interface.lvclass"=w4209, "Channel in"=w4194) -> ("error out"=w4216:errorcluster, "Channel out"=w4217:refnum<class "Channel.lvclass">)  [unwired: 7 in]
                    n2179 = call "Write section_name.vi"("error in (no error)"=w4216, "section_name"="CCD_ACS3", "Channel in"=w4217) -> ("error out"=w4214:errorcluster, "Channel out"=w4220:refnum<class "Channel.lvclass">)  [unwired: 7 in]
                    n2180 = call-dynamic "save config.vi"("error in (no error)"=w4214, "file config"="lastsaved.cfg", "Channel in"=w4220) -> ("error out"=w4215:errorcluster, "Channel out"=w4221:refnum<class "Channel.lvclass">)  [unwired: 7 in]
                    n2181 = call-dynamic "Read State Machine.vi"("error in (no error)"=w4215, "Device in"=w4221) -> ("error out"=w4211:errorcluster, "State Machine.lvclass"=w4223:refnum<class "State Machine.lvclass">, "Device out"=w4222:refnum<class "Channel.lvclass">)  [unwired: 7 in]
                    n2182 = call-dynamic "Write State.vi"("error in (no error)"=w4211, "State"=60, "State Machine in"=w4223) -> ("error out"=w4212:errorcluster, "State Machine out"=w4224:refnum<class "State Machine.lvclass">)  [unwired: 7 in]
                    n2183 = call-dynamic "Write State Machine.vi"("error in (no error)"=w4212, "State Machine.lvclass"=w4224, "Device in"=w4222) -> ("error out"=w4226:errorcluster, "Device out"=w4225:refnum<class "Channel.lvclass">)  [unwired: 7 in]
                    n2184 = call-dynamic "Write Channel.vi"("error in (no error)"=w4226, "Channel.lvclass"=w4225, "Acquisition in"=w4195) -> ("error out"=w4190:errorcluster, "Acquisition out"=w4191:refnum<class "Acquisition.lvclass">)  [unwired: 7 in]
                  }
                }
                n2185 = case shown="True" w4137 {
                  tunnel: w4139 -> [w4150 w4154]
                  tunnel: w4138 -> [w4149 w4153]
                  tunnel: [w4150 w4152] -> w4117
                  tunnel: [w4149 w4151] -> w4116
                  frame False {
                  }
                  frame True {
                    # "Ext Start"
                    # "nome do arquivo .cfg"
                    # "seção no arquivo .cfg"
                    n2186 = call-dynamic "Read Channel.vi"("error in (no error)"=w4153, "Acquisition in"=w4154) -> ("error out"=w4184:errorcluster, "Channel.lvclass"=w4185:refnum<class "Channel.lvclass">, "Acquisition out"=w4186:refnum<class "Acquisition.lvclass">)  [unwired: 7 in]
                    n2187 = call-dynamic "Read Interface.vi"("error in (no error)"=w4184, "Channel in"=w4185) -> ("error out"=w4176:errorcluster, "Interface.lvclass"=w4175:refnum<class "Interface.lvclass">, "Channel out"=w4187:refnum<class "Channel.lvclass">)  [unwired: 7 in]
                    n2188 = call-dynamic "Get CCD_Config.vi"("error in (no error)"=w4176, "Interface in"=w4175) -> ("error out"=w4179:errorcluster, "output cluster"=w4180:T31, "Interface out"=w4174:refnum<class "Interface.lvclass">)  [unwired: 7 in]
                    n2189 = Bundle By Name(cluster=w4180, "TRIGGER_MODE"=u8 6 ("SHUTTER_MODE")) -> (w4178:T31)
                    n2190 = call-dynamic "Set CCD_Config.vi"("error in (no error)"=w4179, "input cluster"=w4178, "Interface in"=w4174) -> ("error out"=w4181:errorcluster, "Interface out"=w4173:refnum<class "Interface.lvclass">)  [unwired: 7 in]
                    n2191 = Flatten To String(anything=w4178, error in (no error)=w4181) -> (data string=w4183:string, error out=w4182:errorcluster)  [unwired: 2 in, 1 out]
                    n2192 = call "Write flatted cluster.vi"("error in (no error)"=w4182, "flatted cluster"=w4183, "Interface in"=w4173) -> ("error out"=w4171:errorcluster, "Interface out"=w4172:refnum<class "Interface.lvclass">)  [unwired: 7 in]
                    n2193 = call-dynamic "Write Interface.vi"("error in (no error)"=w4171, "Interface.lvclass"=w4172, "Channel in"=w4187) -> ("error out"=w4165:errorcluster, "Channel out"=w4164:refnum<class "Channel.lvclass">)  [unwired: 7 in]
                    n2194 = call "Write section_name.vi"("error in (no error)"=w4165, "section_name"="CCD_ACS4", "Channel in"=w4164) -> ("error out"=w4167:errorcluster, "Channel out"=w4161:refnum<class "Channel.lvclass">)  [unwired: 7 in]
                    n2195 = call-dynamic "save config.vi"("error in (no error)"=w4167, "file config"="lastsaved.cfg", "Channel in"=w4161) -> ("error out"=w4166:errorcluster, "Channel out"=w4160:refnum<class "Channel.lvclass">)  [unwired: 7 in]
                    n2196 = call-dynamic "Read State Machine.vi"("error in (no error)"=w4166, "Device in"=w4160) -> ("error out"=w4170:errorcluster, "State Machine.lvclass"=w4158:refnum<class "State Machine.lvclass">, "Device out"=w4159:refnum<class "Channel.lvclass">)  [unwired: 7 in]
                    n2197 = call-dynamic "Write State.vi"("error in (no error)"=w4170, "State"=60, "State Machine in"=w4158) -> ("error out"=w4169:errorcluster, "State Machine out"=w4157:refnum<class "State Machine.lvclass">)  [unwired: 7 in]
                    n2198 = call-dynamic "Write State Machine.vi"("error in (no error)"=w4169, "State Machine.lvclass"=w4157, "Device in"=w4159) -> ("error out"=w4155:errorcluster, "Device out"=w4156:refnum<class "Channel.lvclass">)  [unwired: 7 in]
                    n2199 = call-dynamic "Write Channel.vi"("error in (no error)"=w4155, "Channel.lvclass"=w4156, "Acquisition in"=w4186) -> ("error out"=w4151:errorcluster, "Acquisition out"=w4152:refnum<class "Acquisition.lvclass">)  [unwired: 7 in]
                  }
                }
                n2200 = call-dynamic "Write AcquisitionA.vi"("error in (no error)"=w4122, "Acquisition.lvclass"=w4123, "S4ACS_GUI in"=w4124) -> ("error out"=w4113:errorcluster, "S4ACS_GUI out"=w4128:refnum<class "S4GUI.lvclass">)  [unwired: 7 in]
                n2201 = call "Write AcquisitionB.vi"("error in (no error)"=w4120, "Acquisition.lvclass"=w4121, "S4ACS_GUI in"=w4128) -> ("error out"=w4112:errorcluster, "S4ACS_GUI out"=w4127:refnum<class "S4GUI.lvclass">)  [unwired: 7 in]
                n2202 = call-dynamic "Write AcquisitionC.vi"("error in (no error)"=w4118, "Acquisition.lvclass"=w4119, "S4ACS_GUI in"=w4127) -> ("error out"=w4111:errorcluster, "S4ACS_GUI out"=w4126:refnum<class "S4GUI.lvclass">)  [unwired: 7 in]
                n2203 = call-dynamic "Write AcquisitionD.vi"("error in (no error)"=w4116, "Acquisition.lvclass"=w4117, "S4ACS_GUI in"=w4126) -> ("error out"=w4110:errorcluster, "S4ACS_GUI out"=w4125:refnum<class "S4GUI.lvclass">)  [unwired: 7 in]
                n2204 = Merge Errors(w4113, w4112, w4111, w4110) -> (w4109:errorcluster)
              }
            }
            n2205 = call-dynamic "Read prev ciclos.vi"("error in (no error)"=w4096, "S4GUI in"=w4097) -> ("error out"=w4094:errorcluster, "prev ciclos"=w4093:u32, "S4GUI out"=w4095:refnum<class "S4GUI.lvclass">)  [unwired: 7 in]
            n2206 = property on="#Cycles Done" class="Slide (strict)"("Scale.Maximum"=w4093, "Scale.Minimum"=0.0 ("Scale.Range:Minimum")) -> ()  [unwired: 2 in, 2 out]
            n2207 = local write "# Cycles"(w4093) -> ()
          }
          frame 0, Default {
            # "Async mode: Os canais são configurados com Trigger Interno para Fotometria ou Trigger Externo para Polarimetria (independentemente do status do SyncBox)"
            # "Aynchronous:"
            n2208 = call-dynamic "Read AcquisitionC.vi"("error in (no error)"=w4328, "S4ACS_GUI in"=w4327) -> ("error out"=w4332:errorcluster, "Acquisition.lvclass"=w4331:refnum<class "Acquisition.lvclass">)  [unwired: 7 in, 1 out]
            n2209 = call "Read AcquisitionB.vi"("error in (no error)"=w4328, "S4ACS_GUI in"=w4327) -> ("error out"=w4333:errorcluster, "Acquisition.lvclass"=w4334:refnum<class "Acquisition.lvclass">)  [unwired: 7 in, 1 out]
            n2210 = call-dynamic "Read AcquisitionA.vi"("error in (no error)"=w4328, "S4ACS_GUI in"=w4327) -> ("error out"=w4335:errorcluster, "Acquisition.lvclass"=w4336:refnum<class "Acquisition.lvclass">, "S4ACS_GUI out"=w4317:refnum<class "S4GUI.lvclass">)  [unwired: 7 in]
            n2211 = case shown="True" w4308 {
              tunnel: [u8 0 ("SHUTTER_MODE") w4351] -> w4307
              tunnel: w4306 -> [_ w4354]
              frame False {
                # "Fotom."
                # "Internal"
              }
              frame True {
                # "exp mode?"
                # "Internal"
                # "Polar."
                # "Ext. Start"
                n2212 = Select(t=u8 0, s=w4354, f=u8 6 ("SHUTTER_MODE")) -> (s? t:f=w4351:u8)
              }
            }
            n2213 = call-dynamic "Read AcquisitionD.vi"("error in (no error)"=w4328, "S4ACS_GUI in"=w4327) -> ("error out"=w4329:errorcluster, "Acquisition.lvclass"=w4330:refnum<class "Acquisition.lvclass">)  [unwired: 7 in, 1 out]
            n2214 = call "Read connection.vi"("error in (no error)"=w4332, "Server in"=w4331) -> ("error out"=w4341:errorcluster, "connection"=w4340:bool, "Server out"=w4342:refnum<class "Acquisition.lvclass">)  [unwired: 7 in]
            n2215 = call "Read connection.vi"("error in (no error)"=w4333, "Server in"=w4334) -> ("error out"=w4344:errorcluster, "connection"=w4343:bool, "Server out"=w4345:refnum<class "Acquisition.lvclass">)  [unwired: 7 in]
            n2216 = call "Read connection.vi"("error in (no error)"=w4329, "Server in"=w4330) -> ("error out"=w4338:errorcluster, "connection"=w4337:bool, "Server out"=w4339:refnum<class "Acquisition.lvclass">)  [unwired: 7 in]
            n2217 = call "Read connection.vi"("error in (no error)"=w4335, "Server in"=w4336) -> ("error out"=w4347:errorcluster, "connection"=w4346:bool, "Server out"=w4348:refnum<class "Acquisition.lvclass">)  [unwired: 7 in]
            n2218 = case shown="True" w4340 {
              tunnel: w4342 -> [w4399 w4410]
              tunnel: w4341 -> [w4398 w4409]
              tunnel: [w4399 w4408] -> w4312
              tunnel: [w4398 w4407] -> w4311
              tunnel: w4307 -> [_ w4406]
              frame False {
              }
              frame True {
                # "nome do arquivo .cfg"
                # "seção no arquivo .cfg"
                n2219 = call-dynamic "Read Channel.vi"("error in (no error)"=w4409, "Acquisition in"=w4410) -> ("error out"=w4414:errorcluster, "Channel.lvclass"=w4413:refnum<class "Channel.lvclass">, "Acquisition out"=w4412:refnum<class "Acquisition.lvclass">)  [unwired: 7 in]
                n2220 = call-dynamic "Read Interface.vi"("error in (no error)"=w4414, "Channel in"=w4413) -> ("error out"=w4421:errorcluster, "Interface.lvclass"=w4422:refnum<class "Interface.lvclass">, "Channel out"=w4411:refnum<class "Channel.lvclass">)  [unwired: 7 in]
